vi "Read Stage Position.vi"(4 "error in":errorcluster, 5 "VISA resource name in":refnum<visa-resource-name>) -> (0 "Current Position":cluster{dbl, dbl, dbl}, 1 "error out":errorcluster, 2 "VISA resource name out":refnum<visa-resource-name>)   [LabVIEW 2014]
uses:
  <vilib>/Instr/_visa.llb/VISA Configure Serial Port (Instr).vi
panel:
  out "Serial Settings:Number of Bytes at Serial Port":u32
  out "read buffer":string
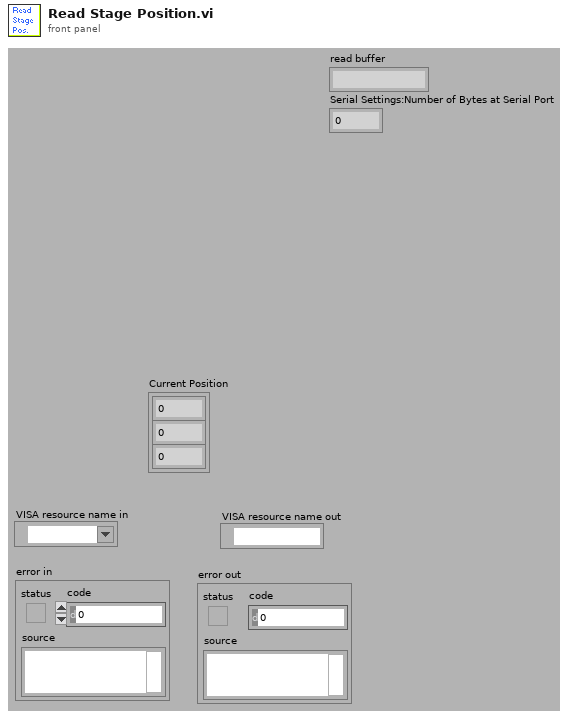
[diagram p1: front panel]
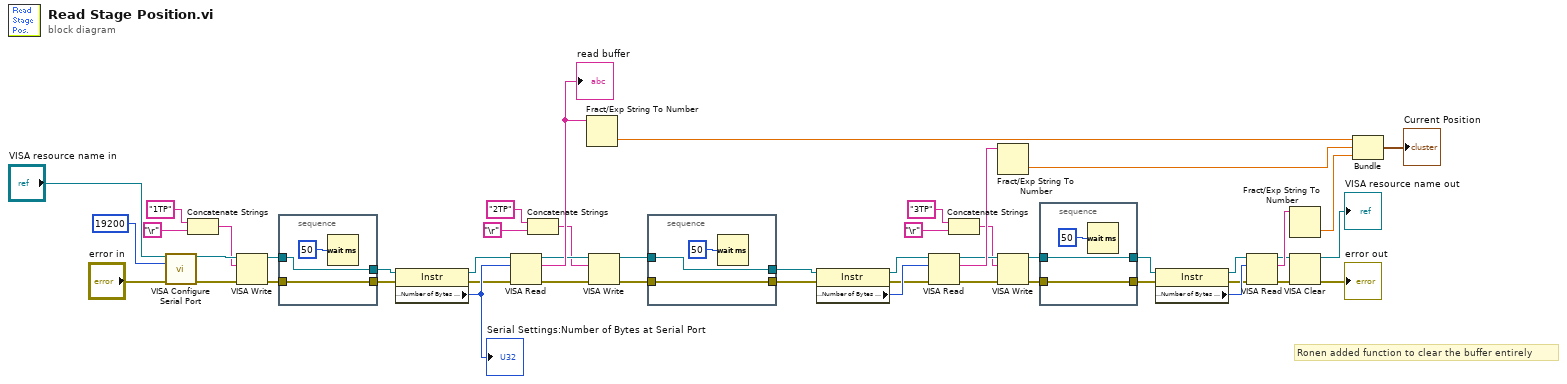
[diagram p0: block diagram]
diagram:
  # "Ronen added function to clear the buffer entirely"
  n1 = call-poly "VISA Configure Serial Port"("VISA resource name"="VISA resource name in", "baud rate (9600)"=u32 19200, "error in (no error)"="error in") -> ("VISA resource name out"=w47:refnum<visa-resource-name>, "error out"=w46:errorcluster)  [unwired: 3 in, 8 out]
  n2 = Concatenate Strings("1TP" ("write buffer"), "\r") -> (w16:string)
  n3 = VISA Write(VISA resource name=w47, write buffer=w16, error in (no error)=w46) -> (VISA resource name out=w45:refnum<visa-resource-name>, error out=w44:errorcluster)  [unwired: 1 out]
  n4 = stacked-sequence {
    tunnel: [w53] -> w43
    tunnel: w45 -> [w53]
    tunnel: w44 -> [w52]
    tunnel: [w52] -> w38
    frame #0 {
      n5 = Wait (ms)(milliseconds to wait=50) -> ()  [unwired: 1 out]
    }
  }
  n6 = property class="Instr"(reference=w43, error in=w38) -> (reference out=w42:refnum<visa-resource-name>, error out=w40:errorcluster, "Serial Settings:Number of Bytes at Serial Port"=w41:u32)
  "Serial Settings:Number of Bytes at Serial Port" <- w41
  n7 = VISA Read(VISA resource name=w42, byte count=w41, error in (no error)=w40) -> (VISA resource name out=w21:refnum<visa-resource-name>, read buffer=w39:string, error out=w19:errorcluster)  [unwired: 1 out]
  "read buffer" <- w39
  n8 = Concatenate Strings("2TP" ("write buffer"), "\r") -> (w15:string)
  n9 = Fract/Exp String To Number(string=w39) -> (number=w11:dbl)  [unwired: 4 out]
  n10 = VISA Write(VISA resource name=w21, write buffer=w15, error in (no error)=w19) -> (VISA resource name out=w37:refnum<visa-resource-name>, error out=w36:errorcluster)  [unwired: 1 out]
  n11 = stacked-sequence {
    tunnel: [w56] -> w35
    tunnel: w37 -> [w56]
    tunnel: w36 -> [w55]
    tunnel: [w55] -> w30
    frame #0 {
      n12 = Wait (ms)(milliseconds to wait=50) -> ()  [unwired: 1 out]
    }
  }
  n13 = property class="Instr"(reference=w35, error in=w30) -> (reference out=w34:refnum<visa-resource-name>, error out=w32:errorcluster, "Serial Settings:Number of Bytes at Serial Port"=w33:u32)
  n14 = VISA Read(VISA resource name=w34, byte count=w33, error in (no error)=w32) -> (VISA resource name out=w20:refnum<visa-resource-name>, read buffer=w31:string, error out=w18:errorcluster)  [unwired: 1 out]
  n15 = Concatenate Strings("3TP" ("write buffer"), "\r") -> (w13:string)
  n16 = Fract/Exp String To Number(string=w31) -> (number=w10:dbl)  [unwired: 4 out]
  n17 = VISA Write(VISA resource name=w20, write buffer=w13, error in (no error)=w18) -> (VISA resource name out=w29:refnum<visa-resource-name>, error out=w28:errorcluster)  [unwired: 1 out]
  n18 = stacked-sequence {
    tunnel: [w59] -> w27
    tunnel: w29 -> [w59]
    tunnel: w28 -> [w58]
    tunnel: [w58] -> w22
    frame #0 {
      n19 = Wait (ms)(milliseconds to wait=50) -> ()  [unwired: 1 out]
    }
  }
  n20 = property class="Instr"(reference=w27, error in=w22) -> (reference out=w26:refnum<visa-resource-name>, error out=w24:errorcluster, "Serial Settings:Number of Bytes at Serial Port"=w25:u32)
  n21 = VISA Read(VISA resource name=w26, byte count=w25, error in (no error)=w24) -> (VISA resource name out=w2:refnum<visa-resource-name>, read buffer=w23:string, error out=w4:errorcluster)  [unwired: 1 out]
  n22 = Fract/Exp String To Number(string=w23) -> (number=w9:dbl)  [unwired: 4 out]
  n23 = VISA Clear(VISA resource name=w2, error in (no error)=w4) -> (VISA resource name out=→"VISA resource name out":refnum<visa-resource-name>, error out=→"error out":errorcluster)
  n24 = Bundle(w11, w10, w9) -> (→"Current Position":cluster{dbl, dbl, dbl})  [unwired: 1 out]
